vi "MPUSBRead.vi"(6 "maxLength":dbl, 7 "dwMilliseconds":u32=1000, 8 "error in (no error)":errorcluster, 9 "pLength":u32, 10 "dwLen":u32=3, 11 "handleIn":u32 format="%x") -> (0 "error out":errorcluster, 1 "pDataOut":u8[](array[numeric]), 2 "return type":u32, 3 "handleOut":u32 format="%x", 4 "setValue":dbl, 5 "cmd":u8)   [LabVIEW 2019]
doc: "// Note that \"input\" and \"output\" refer to the parameter designations in calls\n// to this function, which are the opposite of common sense from the\n// perspective of an application making the calls.\n//\nDWORD MPUSBRead(HANDLE handle, // Input\n PVOID pData, // Output\n DWORD dwLen, // Input\n PDWORD pLength, // Output\n DWORD dwMilliseconds); // Input\n\nWritten by: Complete Automated Solutions\nwww.CompleteAutomatedSolutions.com"
uses:
  mpusbapi.dll
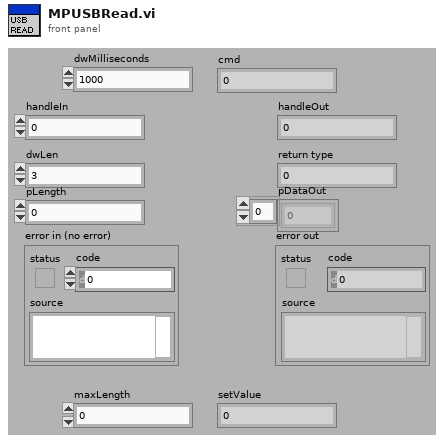
[diagram p1: front panel]
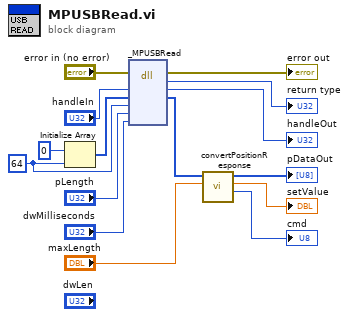
[diagram p0: block diagram]
diagram:
  w9 = 64
  n1 = Initialize Array(u8 0, w9) -> (w10:u8[])
  n2 = dll-call lib="C:/Users/z003r4zd/Desktop/Point Contact Mods 2019/Automation/Actuonix/LAC+Labview+Example/Actuonix_LAC_LabVIEW_Example/USB_VIs/mpusbapi.dll" fn="_MPUSBRead"(error in="error in (no error)", "handle"="handleIn", "pData"=w10, "dwLen"=w9, "pLength"="pLength", "dwMilliseconds"="dwMilliseconds") -> (error out=→"error out":errorcluster, "return type"=→"return type":u32, "handle"=→"handleOut":u32, "pData"=w5:u8[])  [unwired: 5 in, 1 out]
  n3 = call "convertPositionResponse.vi"("maxLength"="maxLength", "pData"=w5) -> ("cmd"=→"cmd":u8, "position"=→"setValue":dbl, "rawDataOut"=→"pDataOut":u8[])  [unwired: 4 in, 3 out]
